vi "Check if ready for next step.vi"(0 "data step cluster":T1, 7 "Time since action":timestamp, 9 "Operator input":bool, 11 "error in (no error)":errorcluster, 13 "User input 1":dbl) -> (4 "Next step":bool, 10 "Show operator button":bool, 15 "error out":errorcluster)   [LabVIEW 2011]
uses:
  Sequence steps config..ctl
  Single criteria cluster.ctl
  Criteria types.ctl
  Boolean operation.ctl
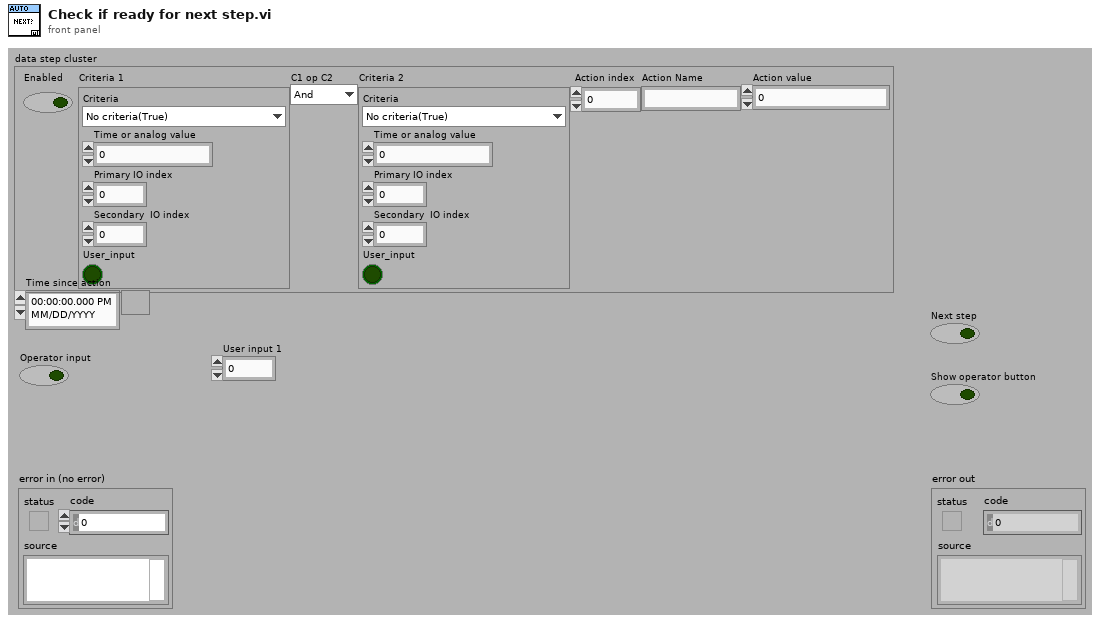
[diagram p1: front panel]
types:
  T1 = typedef "Sequence steps config..ctl" = cluster{"Enabled":bool, "Criteria 1":T2, "C1 op C2":T4, "Criteria 2":T2, "Action index":i32, "Action Name":string, "Action value":dbl}
  T2 = typedef "Single criteria cluster.ctl" = cluster{"Criteria":T3, "Time or analog value":dbl, "Primary IO index":i32, "Secondary  IO index":i32, "User_input":bool}
  T3 = typedef "Criteria types.ctl" = enum16{"No criteria(True)", "Time(s)", "Analog IO over", "Analog IO over or equal", "Analog IO under", "Analog IO under or equal", "Analog IO 1 minus Analog IO 2 over", "Digital IO True", "Digital IO False", "Operator approval"}
  T4 = typedef "Boolean operation.ctl" = enum16{"And", "Or", "Xor", "Nand", "Nor", "Nxor", "Implies"}
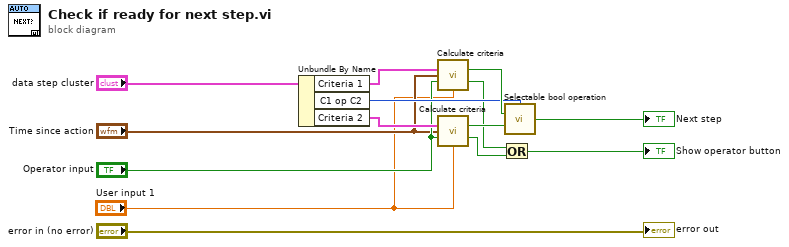
[diagram p0: block diagram]
diagram:
  n1 = Unbundle By Name("data step cluster") -> ("Criteria 1"=w7:T2, "C1 op C2"=w9:T4, "Criteria 2"=w8:T2)
  n2 = call "Calculate criteria.vi"("Criteria"=w7, "Sequence step started"="Time since action", "Operator presse OK"="Operator input", "User input 1"="User input 1") -> ("Continue"=w10:bool, "Show opperator aproval  button"=w2:bool)  [unwired: 9 in, 1 out]
  n3 = call "Calculate criteria.vi"("Criteria"=w8, "Sequence step started"="Time since action", "Operator presse OK"="Operator input", "User input 1"="User input 1") -> ("Continue"=w11:bool, "Show opperator aproval  button"=w12:bool)  [unwired: 9 in, 1 out]
  n4 = Or(x=w2, y=w12) -> (x .or. y?=→"Show operator button":bool)
  n5 = call "Selectable bool operation.vi"("Criteria boolean operation"=w9, "Criteria x"=w10, "Criteria y"=w11) -> ("x bool operation y."=→"Next step":bool)  [unwired: 12 in]
  "error out" <- "error in (no error)"
